vi "Utility - Read RS485.vi"(8 "error in":errorcluster caption="错误输入（无错误）", 11 "VISA resource name":refnum<visa-resource-name>="COM2") -> (0 "error out":errorcluster caption="错误输出")   [LabVIEW 2015]
uses:
  <vilib>/Instr/_visa.llb/VISA Configure Serial Port (Instr).vi
panel:
  out "读取缓冲区":string
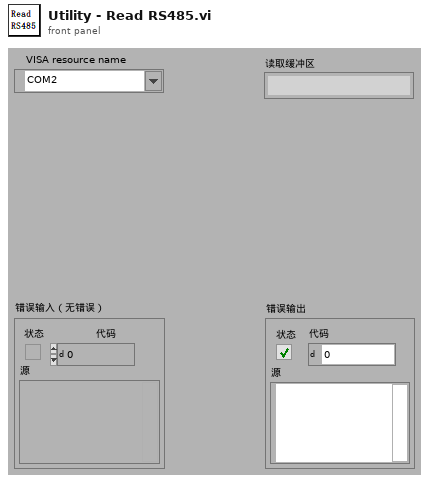
[diagram p1: front panel]
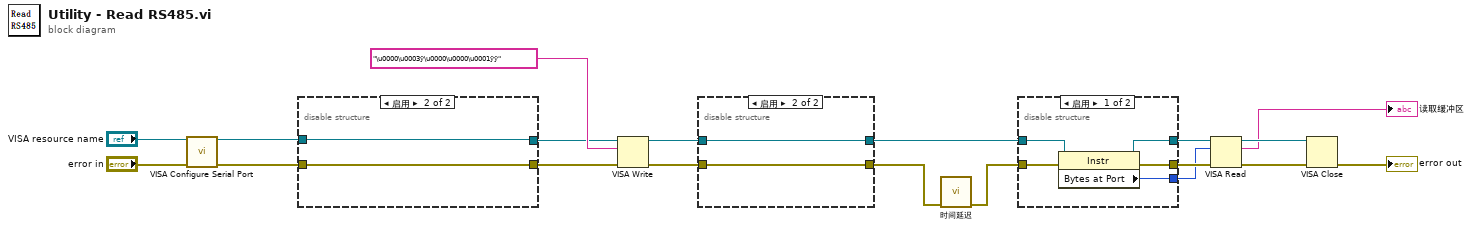
[diagram p0: block diagram]
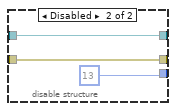
[diagram p2: hidden frame]
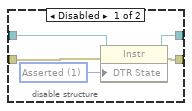
[diagram p3: hidden frame]
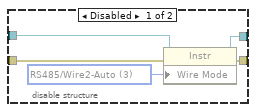
[diagram p4: hidden frame]
diagram:
  n1 = call-poly "VISA Configure Serial Port"("VISA resource name"="VISA resource name", "error in (no error)"="error in") -> ("VISA resource name out"=w6:refnum<visa-resource-name>, "error out"=w13:errorcluster)  [unwired: 12 in]
  n2 = disable-structure shown="启用" {
    disable-tunnel: w6 -> [w24 w26]
    disable-tunnel: w13 -> [w22 w25]
    disable-tunnel: [w21 w26] -> w11
    disable-tunnel: [w20 w25] -> w12
    frame Disabled {
      w23 = i16 3 items=["Unknown"=-1, "RS485/Wire4"=0, "RS485/Wire2-EchoDTR"=1, "RS485/Wire2-CtrlDTR"=2, "RS485/Wire2-Auto"=3, "RS232/DTE"=128, "RS232/DCE"=129, "RS232/AUTO"=130] ("Serial Settings:Wire Mode")
      n3 = property class="Instr"(reference=w24, error in=w22, "Wire Mode"=w23) -> (reference out=w21:refnum<visa-resource-name>, error out=w20:errorcluster)
    }
    frame Enabled {
    }
  }
  n4 = VISA Write(VISA resource name=w11, write buffer="\u0000\u0003ÿ\u0000\u0000\u0001ÿÿ" ("写入缓冲区"), error in (no error)=w12) -> (VISA resource name out=w10:refnum<visa-resource-name>, error out=w8:errorcluster)  [unwired: 1 out]
  n5 = disable-structure shown="启用" {
    disable-tunnel: w10 -> [w31 w33]
    disable-tunnel: [w30 w33] -> w9
    disable-tunnel: w8 -> [w28 w32]
    disable-tunnel: [w27 w32] -> w7
    frame Disabled {
      w29 = i16 1 items=["Unknown"=-1, "Unasserted"=0, "Asserted"=1] ("Serial Settings:Modem Line Settings:Line DTR State")
      n6 = property class="Instr"(reference=w31, error in=w28, "DTR State"=w29) -> (reference out=w30:refnum<visa-resource-name>, error out=w27:errorcluster)
    }
    frame Enabled {
    }
  }
  n7 = call "时间延迟"("error in (no error)"=w7) -> ("error out"=w1:errorcluster)  [unwired: 10 in]
  n8 = disable-structure shown="启用" {
    disable-tunnel: w9 -> [w38 w41]
    disable-tunnel: [w37 w41] -> w4
    disable-tunnel: [w36 w40] -> w3
    disable-tunnel: w1 -> [w35 w40]
    disable-tunnel: [w34 u32 13 ("Bytes at Port")] -> w2
    frame Enabled {
      n9 = property class="Instr"(reference=w38, error in=w35) -> (reference out=w37:refnum<visa-resource-name>, error out=w36:errorcluster, "Bytes at Port"=w34:u32)
    }
    frame Disabled {
    }
  }
  n10 = VISA Read(VISA resource name=w4, byte count=w2, error in (no error)=w3) -> (VISA resource name out=w18:refnum<visa-resource-name>, read buffer=→"读取缓冲区":string, error out=w17:errorcluster)  [unwired: 1 out]
  n11 = VISA Close(VISA resource name=w18, error in (no error)=w17) -> (error out=→"error out":errorcluster)
